vi "RTMain.vi"() -> ()   [LabVIEW 2013]
uses:
  FPGA/FPGATargetClass/FPGATarget.lvclass
  FPGA/TriggerBoxCalls/TriggerBox.lvclass
  <vilib>/userdefined/High Color/nirio_resource_hc.ctl
  TrigBoxIniFileClass/TrigBoxINIFileClass.lvclass
  <vilib>/Platform/TimedLoop/XDataNode/timing_clust.ctl
  <vilib>/Platform/TimedLoop/XDataNode/nitl_modes.ctl
  <vilib>/Platform/TimedLoop/XDataNode/wakeup.ctl
  <vilib>/event_ctls.llb/usereventprio.ctl
  <vilib>/platform/TimedLoop/XDataNode/XDataNode.xnode
  <vilib>/Platform/TimedLoop/XDataNode/XDNodeRunTimeDep.lvlib
panel:
  in  "STOP":bool
  out "CONNECTING":bool
  out "UDP_OK":bool
  out "FPGA_OK":bool
  out "errorOut":errorcluster
  out "Trigger":bool
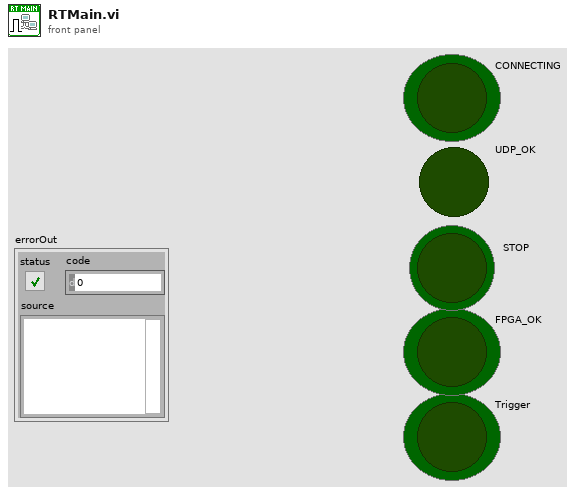
[diagram p1: front panel]
types:
  T1 = typedef "nirio_resource_hc.ctl" = tag
  T2 = typedef "XDNodeRunTimeDep.lvlib/timing_clust.ctl" = cluster{"Expected End [f-1]":u64, "Actual End [f-1]":u64, "Finished Late? [f-1]":bool, "Expected End [i-1]":u64, "Actual End [i-1]":u64, "Finished Late? [i-1]":bool, "Expected Start [i]":u64, "Actual Start [i]":u64, "Expected Start [f]":u64, "Actual Start [f]":u64, "Source Name":string, "Structure Name":string, "Period":i64, "Deadline":i64, "Offset":i64, "Start":i64, "Priority":i32, "Timeout":i32, "Mode":T3, "Wakeup Reason":T4, "Error":errorcluster, "Source Type":string, "Secondary Source Type":string, "Global End Time":u64, "Global Start Time":u64, "Frame Duration":u64, "Iteration Duration":u64, "Assigned CPU":i32, "I/O Scan Engine Mode":u32}
  T3 = typedef "XDNodeRunTimeDep.lvlib/nitl_modes.ctl" = enum32{"No Change", "Process missed periods, maintain original phase", "Discard missed periods, maintain original phase", "Process missed periods, ignore original phase", "Discard missed periods, ignore original phase"}
  T4 = typedef "XDNodeRunTimeDep.lvlib/wakeup.ctl" = enum32{"Normal", "Aborted", "Asynchronous wakeup", "Timing source error", "Timed loop error", "Timeout"}
  T5 = typedef "usereventprio.ctl" = enum32{"high priority", "normal priority"}
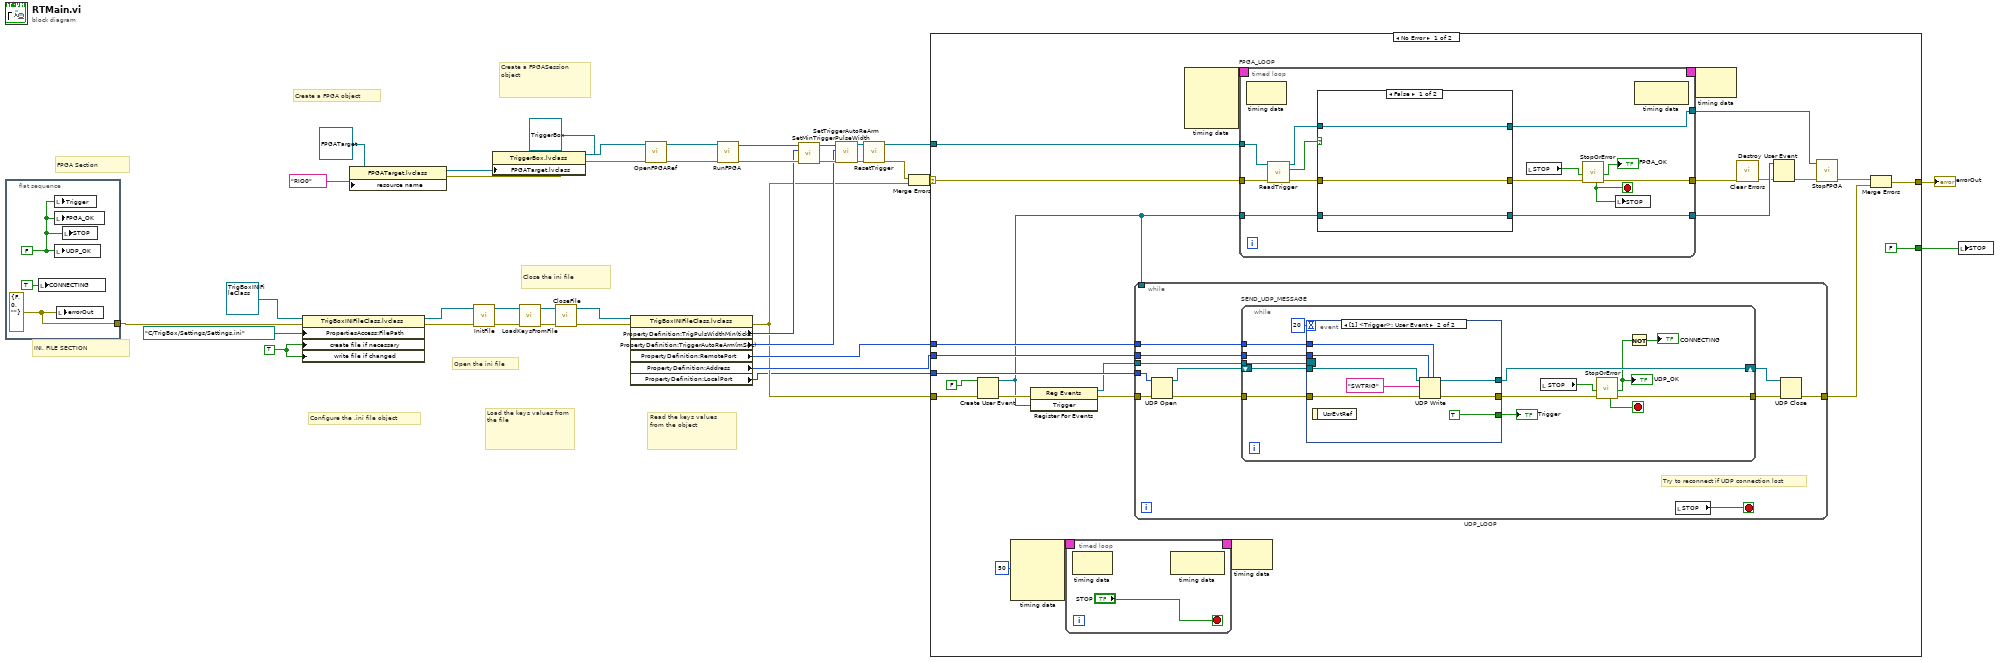
[diagram p0: block diagram]
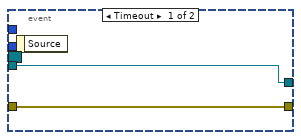
[diagram p2: hidden frame]
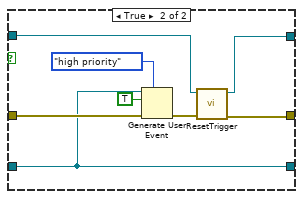
[diagram p3: hidden frame]
diagram:
  w18 = TRUE ("create file if necessary")
  # "INI. FILE SECTION"
  # "FPGA Section"
  # "Read the keys values from the object"
  # "Close the ini file"
  # "Configure the .ini file object"
  # "Load the keys values from the file"
  # "Open the ini file"
  # "Create a FPGASession object"
  # "Create a FPGA object"
  n1 = flat-sequence {
    tunnel: [w40] -> w2
    frame #0 {
      w39 = FALSE ("UDP_OK")
      w40 = errorcluster {"status"=FALSE, "code"=0, "source"=""} ("errorOut")
      n2 = local write "CONNECTING"(TRUE ("CONNECTING")) -> ()
      n3 = local write "Trigger"(w39) -> ()
      n4 = local write "FPGA_OK"(w39) -> ()
      n5 = local write "UDP_OK"(w39) -> ()
      n6 = local write "errorOut"(w40) -> ()
      n7 = local write "STOP"(w39) -> ()
    }
  }
  n8 = property class="TrigBoxINIFileClass.lvclass"(reference=refnum<class "TrigBoxINIFileClass.lvclass"> refnum ("TrigBoxINIFileClass.lvclass"), error in=w2, "PropertiesAccess:FilePath"=path "C:/TrigBox/Settings/Settings.ini" ("file path (use dialog)"), "create file if necessary"=w18, "write file if changed"=w18) -> (reference out=w21:refnum<class "TrigBoxINIFileClass.lvclass">, error out=w20:errorcluster)
  n9 = property class="FPGATarget.lvclass"(reference=refnum<class "FPGATarget.lvclass"> refnum ("FPGATarget.lvclass"), "resource name"=T1 "RIO0") -> (reference out=w32:refnum<class "FPGATarget.lvclass">, error out=w30:errorcluster)  [unwired: 1 in]
  n10 = call-dynamic "InitFile.vi"("error in"=w20, "INIFileClass in"=w21) -> ("error out"=w16:errorcluster, "INIFileClass out"=w17:refnum<class "TrigBoxINIFileClass.lvclass">)  [unwired: 8 in]
  n11 = property class="TriggerBox.lvclass"(reference=refnum<class "TriggerBox.lvclass"> refnum ("HWTriggerDetector.lvclass"), error in=w30, "FPGATarget.lvclass"=w32) -> (reference out=w38:refnum<class "TriggerBox.lvclass">, error out=w37:errorcluster)
  n12 = call-dynamic "LoadKeysFromFile.vi"("error in (no error)"=w16, "TrigBoxINIFileClass in"=w17) -> ("error out"=w14:errorcluster, "TrigBoxINIFileClass out"=w15:refnum<class "TrigBoxINIFileClass.lvclass">)  [unwired: 8 in]
  n13 = call-dynamic "CloseFile.vi"("error in (no error)"=w14, "INIFileClass in"=w15) -> ("error out"=w10:errorcluster, "INIFileClass out"=w13:refnum<class "TrigBoxINIFileClass.lvclass">)  [unwired: 7 in, 1 out]
  n14 = property class="TrigBoxINIFileClass.lvclass"(reference=w13, error in=w10) -> (error out=w3:errorcluster, "PropertyDefinition:TrigPulsWidthMin(ticks)"=w12:u64, "PropertyDefinition:TriggerAutoReArm(mSec)"=w11:i64, "PropertyDefinition:RemotePort"=w9:u16, "PropertyDefinition:Address"=w5:u32, "PropertyDefinition:LocalPort"=w1:u32)  [unwired: 1 out]
  n15 = call-dynamic "OpenFPGARef.vi"("error in"=w37, "FPGASession in"=w38) -> ("error out"=w29:errorcluster, "FPGASession out"=w28:refnum<class "TriggerBox.lvclass">)  [unwired: 8 in]
  n16 = call-dynamic "RunFPGA.vi"("error in"=w29, "FPGASession in"=w28) -> ("error out"=w25:errorcluster, "FPGASession out"=w26:refnum<class "TriggerBox.lvclass">)  [unwired: 8 in]
  n17 = call-dynamic "SetMinTriggerPulseWidth.vi"("error in"=w25, "TrigPulsWidthMin(ticks)"=w12, "TriggerBox in"=w26) -> ("error out"=w24:errorcluster, "TriggerBox out"=w23:refnum<class "TriggerBox.lvclass">)  [unwired: 7 in]
  n18 = call-dynamic "SetTriggerAutoReArm.vi"("error in"=w24, "TriggerAutoReArm(mSec)"=w11, "TriggerBox in"=w23) -> ("error out"=w35:errorcluster, "TriggerBox out"=w34:refnum<class "TriggerBox.lvclass">)  [unwired: 7 in]
  n19 = call-dynamic "ResetTrigger.vi"("error in"=w35, "TriggerBox in"=w34) -> ("error out"=w8:errorcluster, "TriggerBox out"=w27:refnum<class "TriggerBox.lvclass">)  [unwired: 8 in]
  n20 = Merge Errors(w8, w3) -> (w7:errorcluster)
  n21 = case shown="No Error" w7 {
    selector: w7 -> [w61 w137]
    tunnel: w27 -> [w62 _]
    tunnel: w9 -> [w54 _]
    tunnel: [w59 w137] -> w6
    tunnel: w3 -> [w46 _]
    tunnel: w5 -> [w52 _]
    tunnel: w1 -> [w53 _]
    tunnel: [FALSE _] -> w4
    frame No Error {
      n22 = Create User Event(user event datatype=FALSE ("Trigger"), error in=w46) -> (user event=w45:refnum<user-event>, error out=w47:errorcluster)
      n23 = node-c288(i64 50 ("Period")) -> (w50:T2)  [unwired: 3 in]
      n24 = register-events(error in=w47, w45) -> (reference out=w43:refnum<event-registration>, error out=w44:errorcluster)  [unwired: 1 in]
      n25 = timed-loop {
        timing: w50 -> [_]
        timing-out: [_] -> w49
        stop <- "STOP" stop-if-true
        n26 = node-c288() -> ()  [unwired: 1 in, 1 out]
        n27 = node-c288() -> ()  [unwired: 1 in, 1 out]
      }
      n28 = while "UDP_LOOP" {
        tunnel: w45 -> [_]
        tunnel: w44 -> [w84]
        tunnel: w54 -> [w83]
        tunnel: w53 -> [w82]
        tunnel: w52 -> [w81]
        tunnel: [w76] -> w51
        tunnel: w43 -> [w74]
        stop <- w79 stop-if-true
        # "Try to reconnect if UDP connection lost"
        n29 = UDP Open(8:w84, 11:w82) -> (port=w80:refnum<k16>, 0:w75:errorcluster)  [unwired: 3 in, 1 out]
        n30 = while "SEND_UDP_MESSAGE" {
          tunnel: w75 -> [w98]
          tunnel: [w91] -> w78
          tunnel: w83 -> [w95]
          tunnel: w81 -> [w88]
          shift-right: [w94] -> w77
          shift-left: w80 -> [w89]
          tunnel: w74 -> [w85]
          stop <- w90 stop-if-true
          n31 = event shown="[1] <Trigger>: User Event" {
            selector: w85 -> [_ _]
            dyn-events: _ -> [_ _]
            timeout: 20 -> [_ _]
            tunnel: w98 -> [w100 w107]
            tunnel: [w100 w106] -> w92
            tunnel: [_ TRUE] -> w97
            tunnel: w95 -> [_ w102]
            tunnel: [w99 w104] -> w94
            tunnel: w89 -> [w99 w103]
            tunnel: w88 -> [_ w101]
            event Timeout {
              n32 = event-data() -> ()  [unwired: 1 in, 1 out]
            }
            event User Event {
              n33 = event-data() -> ()  [unwired: 1 in, 1 out]
              n34 = UDP Write(address=w101, port or service name=w102, connection ID=w103, data in="SWTRIG", 8:w107) -> (error out=w106:errorcluster, 3:w104:refnum<k16>)  [unwired: 1 in]
            }
          }
          "Trigger" <- w97
          n35 = local read "STOP"() -> (w93:bool)
          n36 = call "StopOrError.vi"("error in"=w92, "StoppedIn"=w93) -> ("error_out"=w91:errorcluster, "!Error"=w86:bool, "StoppedOut"=w90:bool)  [unwired: 7 in]
          "UDP_OK" <- w86
          n37 = Not(x=w86) -> (.not. x?=→"CONNECTING":bool)
        }
        n38 = local read "STOP"() -> (w79:bool)
        n39 = UDP Close(connection ID=w77, 8:w78) -> (error out=w76:errorcluster)  [unwired: 1 out]
      }
      n40 = node-c288() -> (w66:T2)  [unwired: 4 in]
      n41 = node-c288(w49) -> ()  [unwired: 1 out]
      n42 = timed-loop "FPGA_LOOP" {
        tunnel: w61 -> [w121]
        tunnel: w62 -> [w120]
        tunnel: w45 -> [w117]
        tunnel: [w109] -> w63
        timing: w66 -> [_]
        timing-out: [_] -> w65
        tunnel: [w114] -> w64
        tunnel: [w116] -> w57
        stop <- w111 stop-if-true
        n43 = node-c288() -> ()  [unwired: 1 in, 1 out]
        n44 = call-dynamic "ReadTrigger.vi"("error in"=w121, "TriggerBox in"=w120) -> ("error out"=w119:errorcluster, "TriggerFired"=w118:bool, "TriggerBox out"=w110:refnum<class "TriggerBox.lvclass">)  [unwired: 6 in, 1 out]
        n45 = case shown="False" w118 {
          tunnel: w119 -> [w125 w134]
          tunnel: [w125 w129] -> w115
          tunnel: w117 -> [w126 w131]
          tunnel: [w126 w131] -> w116
          tunnel: w110 -> [w124 w128]
          tunnel: [w124 w127] -> w109
          frame False {
          }
          frame True {
            n46 = Generate User Event(priority (normal)=usereventprio."high priority", user event=w131, event data cluster=TRUE ("event data"), error in=w134) -> (error out=w130:errorcluster)  [unwired: 1 out]
            n47 = call-dynamic "ResetTrigger.vi"("error in"=w130, "TriggerBox in"=w128) -> ("error out"=w129:errorcluster, "TriggerBox out"=w127:refnum<class "TriggerBox.lvclass">)  [unwired: 8 in]
          }
        }
        n48 = local read "STOP"() -> (w112:bool)
        n49 = call "StopOrError.vi"("error in"=w115, "StoppedIn"=w112) -> ("error_out"=w114:errorcluster, "!Error"=→"FPGA_OK":bool, "StoppedOut"=w111:bool)  [unwired: 7 in]
        n50 = local write "STOP"(w111) -> ()
        n51 = node-c288() -> ()  [unwired: 1 in, 1 out]
      }
      n52 = node-c288(w65) -> ()  [unwired: 1 out]
      n53 = call <vilib>:"Clear Errors.vi"("error in (no error)"=w64) -> ("error out"=w56:errorcluster)  [unwired: 6 in]
      n54 = Destroy User Event(user event=w57, error in=w56) -> (error out=w58:errorcluster)
      n55 = call-dynamic "StopFPGA.vi"("error in"=w58, "FPGASession in"=w63) -> ("error out"=w60:errorcluster)  [unwired: 8 in, 1 out]
      n56 = Merge Errors(w60, w51) -> (w59:errorcluster)
    }
    frame Error {
    }
  }
  "errorOut" <- w6
  n57 = local write "STOP"(w4) -> ()
